vi "Init.vi"(10 "jettl":refnum<class "jettl.lvclass">) -> (3 "Last Ack Msg Strategy out":refnum<class "Last Ack Msg Strategy.lvclass">)   [LabVIEW 2021, in "jettl.lvlib" / "Last Ack Msg Strategy.lvlib" / "Last Ack Msg Strategy.lvclass"]
uses:
  Last Ack Msg Strategy.lvclass
  jettl/jettl.lvclass
  Last Ack Msg Strategy.lvclass/Last Ack Msg Strategy.ctl
  Sender/Sender.lvlib
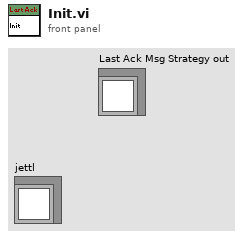
[diagram p1: front panel]
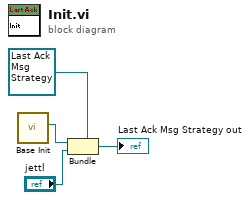
[diagram p0: block diagram]
diagram:
  n1 = call "Base Init.vi"() -> ("Sender"=w1:refnum<class "Sender.lvclass">)  [unwired: 11 in]
  n2 = Bundle "Bundle"(cluster=refnum<class "Last Ack Msg Strategy.lvclass"> refnum ("Last Ack Creator Queue Msg Strategy out"), w1, "jettl") -> (→"Last Ack Msg Strategy out":refnum<class "Last Ack Msg Strategy.lvclass">)
